vi "ECDLesen_ECD.vi"(1 "string":string, 3 "Zwischenspeicher":string[](array[string]), 4 "Port":i32) -> (5 "ECDMW":dbl[](array[numeric]), 7 "Zwischenspeicher":string[](array[string]), 8 "ECDEmpfangen?":bool)   [LabVIEW 2017]
uses:
  <vilib>/regexp/Match Regular Expression.xnode
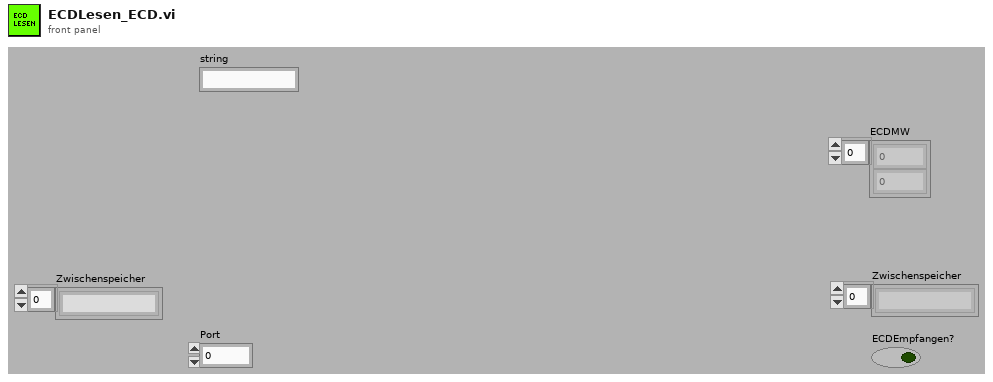
[diagram p1: front panel]
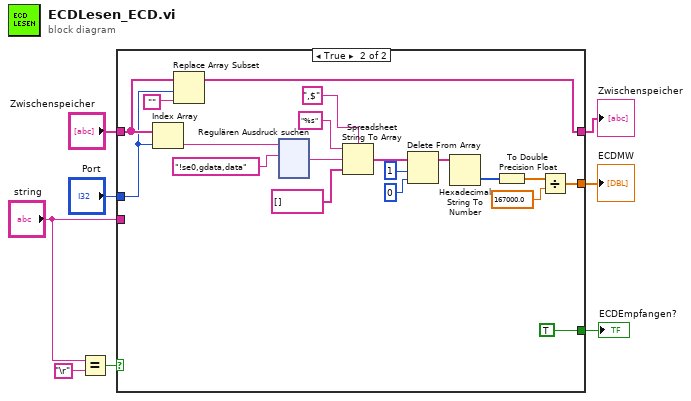
[diagram p0: block diagram]
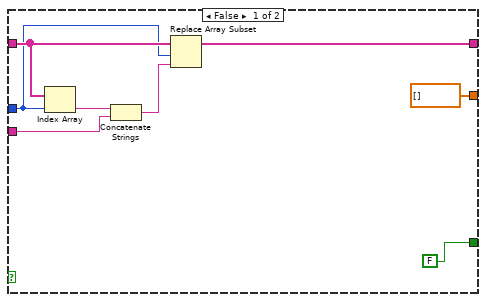
[diagram p2: hidden frame]
diagram:
  n1 = Equal?(x="string", y="\r") -> (x = y?=w7:bool)
  n2 = case shown="True" w7 {
    tunnel: "string" -> [w15 _]
    tunnel: "Zwischenspeicher" -> [w14 w35]
    tunnel: "Port" -> [w13 w34]
    tunnel: [w11 w32] -> w6
    tunnel: [dbl[] [] w18] -> w2
    tunnel: [FALSE TRUE] -> w1
    frame False {
      n3 = Index Array(array=w14, index=w13) -> (element=w16:string)
      n4 = Concatenate Strings(w16, w15) -> (w12:string)
      n5 = Replace Array Subset(array=w14, new element=w12, index=w13) -> (w11:string[])
    }
    frame True {
      n6 = Index Array(array=w35, index=w34) -> (element=w20:string)
      n7 = Replace Array Subset(array=w35, new element="", index=w34) -> (w32:string[])
      n8 = xnode "Regulären Ausdruck suchen"("Eingangs-String"=w20, "Regulärer Ausdruck"="!se0,gdata,data") -> ("Nach Übereinstimmung"=w19:string)  [unwired: 4 in, 4 out]
      n9 = Spreadsheet String To Array(delimiter (Tab)=",$" ("Trennzeichen (Tabulator)"), format string="%s" ("Format-String"), spreadsheet string=w19, array type (2D Dbl)=string[] []) -> (array=w27:string[])
      n10 = Delete From Array(array=w27, length=1 ("Länge"), index=0 ("Index")) -> (array with subset deleted=w24:string[])  [unwired: 1 out]
      n11 = Hexadecimal String To Number(string=w24) -> (number=w23:u32[])  [unwired: 2 in, 1 out]
      n12 = To Double Precision Float(number=w23) -> (double precision float=w22:dbl[])
      n13 = Divide(x=w22, y=167000.0) -> (x/y=w18:dbl[])
    }
  }
  "Zwischenspeicher" <- w6
  "ECDMW" <- w2
  "ECDEmpfangen?" <- w1
